vi "Drive Train Log.vi"   [LabVIEW 2016]
types:
  T1 = typedef "WPI_MotorControlDeviceRef.ctl" = cluster{"DeviceStatus":errorcluster, "Type":T2, "PWM":cluster{"PWM Channel":T3, "DeadBand":T4}, "CAN":cluster{"Device Number":u8, "SetOutput VI Ref":variant, "GetOutput VI Ref":variant, "Enable VI Ref":variant, "Disable VI Ref":variant, "Data":variant}, "Invert":bool}
  T2 = typedef "WPI_MotorControlType.ctl" = enum16{"PWM", "CAN"}
  T3 = typedef "FPGA_DIOPWMChannel.ctl" = enum8{"PWM 0", "PWM 1", "PWM 2", "PWM 3", "PWM 4", "PWM 5", "PWM 6", "PWM 7", "PWM 8", "PWM 9", "PWM MXP 0", "PWM MXP 1", "PWM MXP 2", "PWM MXP 3", "PWM MXP 4", "PWM MXP 5", "PWM MXP 6", "PWM MXP 7", "PWM MXP 8", "PWM MXP 9", "Invalid"}
  T4 = typedef "WPI_PWMDeadband.ctl" = cluster{"Name":string, "maxPositivePwm":i32, "minPositivePwm":i32, "centerPwm":i32, "maxNegativePwm":i32, "minNegativePwm":i32, "angularRange":u16}
  T5 = typedef "WPI_CANTalonSRX_GlobalStatus.ctl" = cluster{"Applied Throttle":dbl, "Module Enabled":bool, "CAN Error":errorcluster, "Closed Loop Error":dbl, "Forward Limit Switch Closed":bool, "Reverse Limit Switch Closed":bool, "Sensor Position":dbl, "Sensor Velocity":dbl, "Current":dbl, "Sticky Fault - Over Temp":bool, "Sticky Fault - Under Voltage":bool, "Sticky Fault - Forward Limit":bool, "Sticky Fault - Reverse Limit":bool, "Sticky Fault - Forward Soft Limit":bool, "Sticky Fault - Reverse Soft Limit":bool, "Brake is Enabled":bool, "Encoder Position":dbl, "Encoder Velocity":dbl, "Encoder Index Count":dbl, "Encoder A Pin State":bool, "Encoder B Pin State":bool, "Encoder Index Pin State":bool, "Analog In":dbl, "Analog In Velocity":dbl, "Temperature (C)":dbl, "Battery Voltage":dbl, "Control 5 Is Supported":bool, "Current Profile Slot Select":dbl, "Pos Div 8":bool, "Vel Div 4":bool, "Pulse Width Position":i32, "Pulse Width Velocity":i32, "Pulse Width Rise To Rise (us)":i32, "Pulse Width Rise To Fall (us)":i32, "Mot Prof Active Is Under Run":bool, "Mot Prof Active Has Under Run":bool, "Mot Prof Active Is Last":bool, "Mot Prof Active Velocity Only":bool, "Mot Prof Active Is Valid":bool, "Mot Prof Buffer Is Full":bool, "Mot Prof Active Profile Slot Select":i32, "Mot Prof NextID":i32, "Mot Prof Count":i32, "Mot Prof Active Velocity":dbl, "Mot Prof Active Position":dbl, "Mot Prof Output Enable":i32}
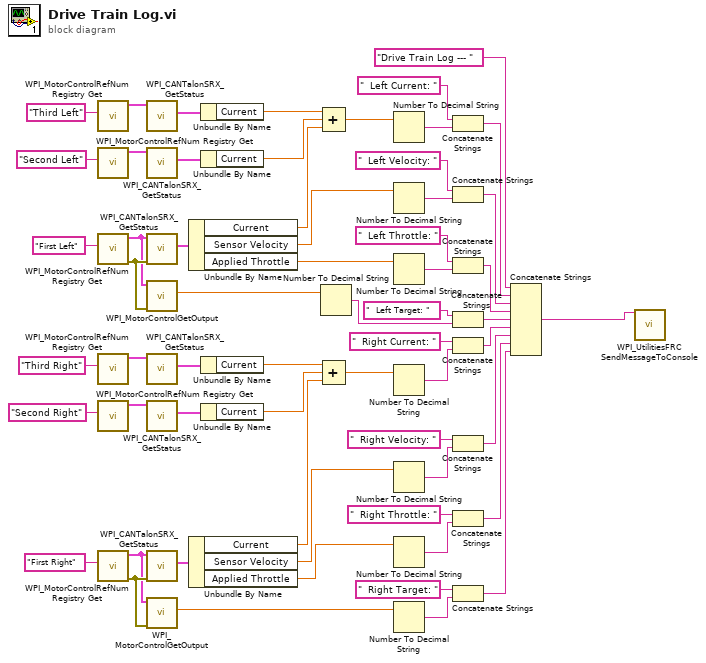
[diagram p0: block diagram]
diagram:
  n1 = call <vilib>:"WPI_MotorControlRefNum Registry Get.vi"("refnum name"="Third Left") -> ("MotorControlDevRef"=w53:T1)  [unwired: 9 in, 1 out]
  n2 = call <vilib>:"WPI_MotorControlRefNum Registry Get.vi"("refnum name"="Second Left") -> ("MotorControlDevRef"=w55:T1)  [unwired: 9 in, 1 out]
  n3 = call <vilib>:"WPI_MotorControlRefNum Registry Get.vi"("refnum name"="First Left") -> ("error out"=w59:errorcluster, "MotorControlDevRef"=w58:T1)  [unwired: 9 in]
  n4 = call <vilib>:"WPI_MotorControlRefNum Registry Get.vi"("refnum name"="Third Right") -> ("MotorControlDevRef"=w40:T1)  [unwired: 9 in, 1 out]
  n5 = call <vilib>:"WPI_MotorControlRefNum Registry Get.vi"("refnum name"="Second Right") -> ("MotorControlDevRef"=w42:T1)  [unwired: 9 in, 1 out]
  n6 = call <vilib>:"WPI_MotorControlRefNum Registry Get.vi"("refnum name"="First Right") -> ("error out"=w46:errorcluster, "MotorControlDevRef"=w45:T1)  [unwired: 9 in]
  n7 = call <vilib>:"WPI_CANTalonSRX_GetStatus.vi"("CAN Talon SRX Ref"=w53) -> ("Talon SRX Status"=w51:T5)  [unwired: 8 in, 2 out]
  n8 = call <vilib>:"WPI_CANTalonSRX_GetStatus.vi"("CAN Talon SRX Ref"=w55) -> ("Talon SRX Status"=w52:T5)  [unwired: 8 in, 2 out]
  n9 = call <vilib>:"WPI_CANTalonSRX_GetStatus.vi"("error in (no error)"=w59, "CAN Talon SRX Ref"=w58) -> ("Talon SRX Status"=w57:T5)  [unwired: 7 in, 2 out]
  n10 = call <vilib>:"WPI_MotorControlGetOutput.vi"("error in"=w59, "MotorControlDevRef"=w58) -> ("Output"=w21:dbl)  [unwired: 7 in, 2 out]
  n11 = call <vilib>:"WPI_CANTalonSRX_GetStatus.vi"("CAN Talon SRX Ref"=w40) -> ("Talon SRX Status"=w38:T5)  [unwired: 8 in, 2 out]
  n12 = call <vilib>:"WPI_CANTalonSRX_GetStatus.vi"("CAN Talon SRX Ref"=w42) -> ("Talon SRX Status"=w39:T5)  [unwired: 8 in, 2 out]
  n13 = call <vilib>:"WPI_CANTalonSRX_GetStatus.vi"("error in (no error)"=w46, "CAN Talon SRX Ref"=w45) -> ("Talon SRX Status"=w44:T5)  [unwired: 7 in, 2 out]
  n14 = call <vilib>:"WPI_MotorControlGetOutput.vi"("error in"=w46, "MotorControlDevRef"=w45) -> ("Output"=w5:dbl)  [unwired: 7 in, 2 out]
  n15 = Unbundle By Name(w57) -> ("Current"=w48:dbl, "Sensor Velocity"=w29:dbl, "Applied Throttle"=w26:dbl)
  n16 = Unbundle By Name(w44) -> ("Current"=w35:dbl, "Sensor Velocity"=w13:dbl, "Applied Throttle"=w9:dbl)
  n17 = Unbundle By Name(w51) -> ("Current"=w49:dbl)
  n18 = Unbundle By Name(w52) -> ("Current"=w50:dbl)
  n19 = Unbundle By Name(w38) -> ("Current"=w36:dbl)
  n20 = Unbundle By Name(w39) -> ("Current"=w37:dbl)
  n21 = Number To Decimal String(number=w21) -> (decimal integer string=w19:string)  [unwired: 1 in]
  n22 = Compound Arithmetic op=ADD(w49, w50, w48) -> (w32:dbl)
  n23 = Compound Arithmetic op=ADD(w36, w37, w35) -> (w17:dbl)
  n24 = Number To Decimal String(number=w32) -> (decimal integer string=w31:string)  [unwired: 1 in]
  n25 = Number To Decimal String(number=w29) -> (decimal integer string=w27:string)  [unwired: 1 in]
  n26 = Number To Decimal String(number=w26) -> (decimal integer string=w25:string)  [unwired: 1 in]
  n27 = Number To Decimal String(number=w17) -> (decimal integer string=w15:string)  [unwired: 1 in]
  n28 = Number To Decimal String(number=w13) -> (decimal integer string=w12:string)  [unwired: 1 in]
  n29 = Number To Decimal String(number=w9) -> (decimal integer string=w8:string)  [unwired: 1 in]
  n30 = Number To Decimal String(number=w5) -> (decimal integer string=w4:string)  [unwired: 1 in]
  n31 = Concatenate Strings("  Left Current: " ("Name"), w31) -> (w30:string)
  n32 = Concatenate Strings("  Left Velocity: " ("Name"), w27) -> (w23:string)
  n33 = Concatenate Strings("  Left Throttle: " ("Name"), w25) -> (w22:string)
  n34 = Concatenate Strings("  Left Target: " ("Name"), w19) -> (w18:string)
  n35 = Concatenate Strings("  Right Current: " ("Name"), w15) -> (w14:string)
  n36 = Concatenate Strings("  Right Velocity: " ("Name"), w12) -> (w10:string)
  n37 = Concatenate Strings("  Right Throttle: " ("Name"), w8) -> (w6:string)
  n38 = Concatenate Strings("  Right Target: " ("Name"), w4) -> (w2:string)
  n39 = Concatenate Strings("Drive Train Log --- " ("string"), w30, w23, w22, w18, w14, w10, w6, w2) -> (w1:string)
  n40 = call <vilib>:"WPI_UtilitiesFRC SendMessageToConsole.vi"("Message"=w1) -> ()  [unwired: 14 in, 1 out]
